vi "List Status Of Source Module.vi"(0 "BroadcastRegistry In":T1, 7 "SourceCSM":string) -> (4 "BroadcastRegistry Out":T1, 6 "Broadcast":string[](array[string]))   [LabVIEW 2017, in "Communicable State Machine.lvlib"]
uses:
  Communicable State Machine.lvlib
  BroadcastRegistry.ctl
  _Shared/CSM Shared.lvlib
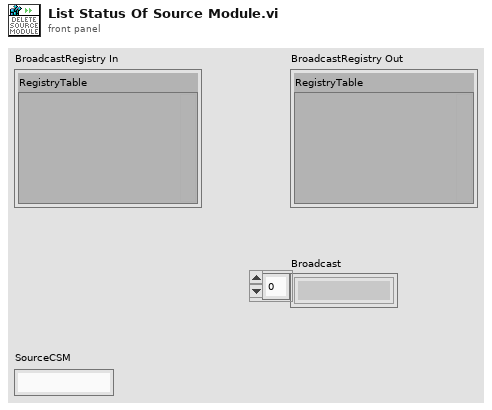
[diagram p1: front panel]
types:
  T1 = typedef "Communicable State Machine.lvlib/BroadcastRegistry.ctl" = cluster{"RegistryTable":variant}
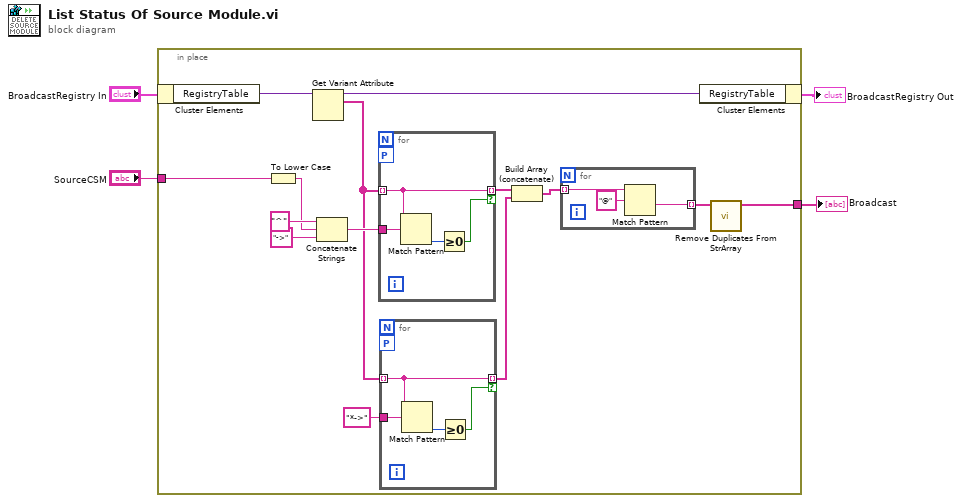
[diagram p0: block diagram]
diagram:
  n1 = in-place {
    in-place-border: "SourceCSM" -> [w12]
    in-place-border: [w9] -> w1
    n2 = in-place-cluster #1("BroadcastRegistry In") -> ("RegistryTable"=w18:variant)
    n3 = To Lower Case(string=w12) -> (all lower case string=w13:string)
    n4 = Get Variant Attribute(Variant=w18) -> (duplicate Variant=w16:variant, names=w8:string[])  [unwired: 3 in, 2 out]
    n5 = Concatenate Strings("^" ("string"), w13, "->" ("string")) -> (w14:string)
    n6 = for {
      tunnel: w8 -> [w29] mode=indexing
      tunnel: [w29] -> w11 mode=indexing if=w26
      tunnel: w14 -> [w28]
      workers-P: _ -> [_]
      n7 = Match Pattern(string=w29, regular expression=w28) -> (offset past match=w27:i32)  [unwired: 1 in, 3 out]
      n8 = Greater Or Equal To 0?(x=w27) -> (x >= 0?=w26:bool)
    }
    n9 = for {
      tunnel: w8 -> [w22] mode=indexing
      tunnel: [w22] -> w5 mode=indexing if=w19
      tunnel: "*->" -> [w21]
      workers-P: _ -> [_]
      n10 = Match Pattern(string=w22, regular expression=w21) -> (offset past match=w20:i32)  [unwired: 1 in, 3 out]
      n11 = Greater Or Equal To 0?(x=w20) -> (x >= 0?=w19:bool)
    }
    n12 = Build Array (concatenate)(w11, w5) -> (w6:string[])
    n13 = for {
      tunnel: w6 -> [w25] mode=indexing
      tunnel: [w23] -> w10 mode=indexing
      n14 = Match Pattern(string=w25, regular expression="@") -> (after substring=w23:string)  [unwired: 1 in, 3 out]
    }
    n15 = in-place-cluster #1("RegistryTable"=w16) -> (→"BroadcastRegistry Out":T1)
    n16 = call "Remove Duplicates From StrArray.vi"("StrArray In"=w10) -> ("StrArray"=w9:string[])  [unwired: 9 in, 1 out]
  }
  "Broadcast" <- w1
